vi "Get Data.vi"(8 "error in":errorcluster, 11 "AlicatCommBank in":refnum<class "AlicatCommBank.lvclass">=refnum) -> (0 "error out":errorcluster, 2 "DataOut":refnum<class "Data.lvclass">[](array[class]), 3 "AlicatCommBank out":refnum<class "AlicatCommBank.lvclass">)   [LabVIEW 2014, in "Alicat.lvlib" / "AlicatCommBank.lvclass"]
doc: "Read the data from the individual controllers. This VI will call <B>Translate Data.vi</B> to turn the data into something meaningful. <B>Translate Data.vi</B> is implemented at the child level."
uses:
  AlicatCommBank.lvclass
  Alicat.lvclass
  Data/MC/AlicatMCData.lvclass
  reusable/Data/Data.lvclass
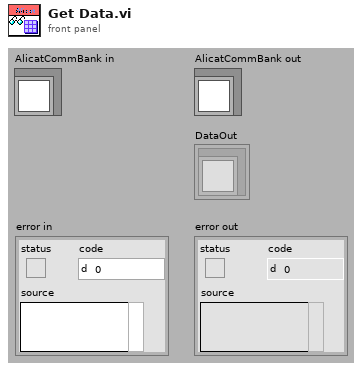
[diagram p1: front panel]
types:
  T1 = cluster{refnum<class "Alicat.lvclass">[], void, void}
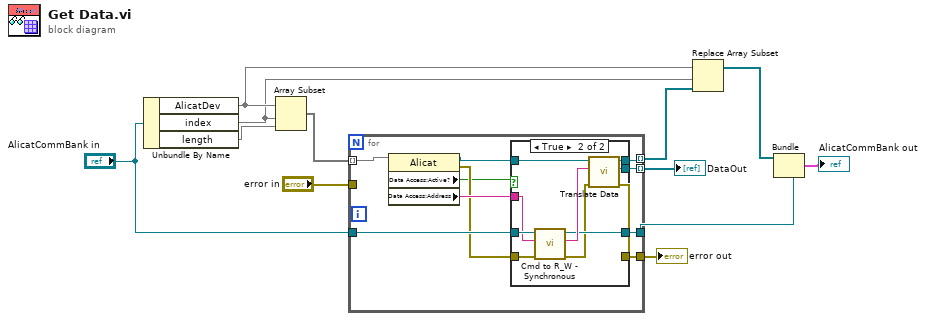
[diagram p0: block diagram]
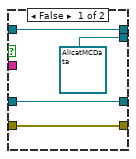
[diagram p2: hidden frame]
diagram:
  n1 = Unbundle By Name("AlicatCommBank in") -> ("AlicatDev"=w3, "index"=w2, "length"=w6)
  n2 = Array Subset(array=w3, index=w2, length=w6) -> (w5:void[])
  n3 = for {
    tunnel: w5 -> [w17] mode=indexing
    tunnel: "AlicatCommBank in" -> [w22]
    tunnel: "error in" -> [_]
    tunnel: [w21] -> w8
    tunnel: [w20] -> w9
    tunnel: [w19] -> w12 mode=indexing
    tunnel: [w18] -> w4 mode=indexing
    n4 = property class="Alicat"(reference=w17) -> (reference out=w16:refnum<class "Alicat.lvclass">, error out=w14:errorcluster, "Data Access:Active?"=w13:bool, "Data Access:Address"=w15:string)  [unwired: 1 in]
    n5 = case shown="True" w13 {
      tunnel: w22 -> [w23 w36]
      tunnel: [w23 w34] -> w21
      tunnel: [w24 w33] -> w20
      tunnel: [refnum<class "AlicatMCData.lvclass"> refnum ("AlicatMData out") w32] -> w19
      tunnel: [w25 w31] -> w18
      tunnel: w16 -> [w25 w29]
      tunnel: w15 -> [_ w28]
      tunnel: w14 -> [w24 w27]
      frame False {
      }
      frame True {
        n6 = call-dynamic "Cmd to R_W - Synchronous.vi"("error in"=w27, "write buffer"=w28, "Serial IO in"=w36) -> ("error out"=w30:errorcluster, "read buffer"=w35:string, "Serial IO out"=w34:refnum<class "AlicatCommBank.lvclass">)  [unwired: 6 in]
        n7 = call-dynamic "Translate Data.vi"("error in (no error)"=w30, "BufferIn"=w35, "Alicat in"=w29) -> ("error out"=w33:errorcluster, "DataOut"=w32:refnum<class "Data.lvclass">, "Alicat out"=w31:refnum<class "Alicat.lvclass">)  [unwired: 6 in]
      }
    }
  }
  "error out" <- w9
  "DataOut" <- w12
  n8 = Replace Array Subset(array=w3, new element=w4, index=w2) -> (w1:refnum<class "Alicat.lvclass">[])
  n9 = Bundle(cluster=w8, w1) -> (→"AlicatCommBank out":T1)  [unwired: 2 in]
